vi "Test Case, Master Record.vi"() -> ()   [LabVIEW 2010]
panel:
  in  "Table Control":string[][](table)
  out "error out":errorcluster
  in  "error in":errorcluster
  in  "Initialize":bool=TRUE
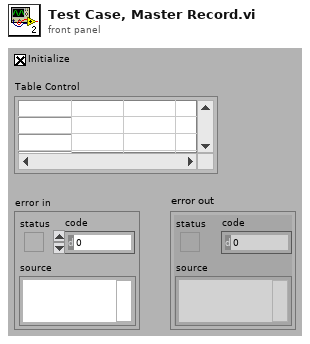
[diagram p1: front panel]
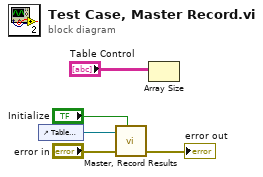
[diagram p0: block diagram]
diagram:
  n1 = control-ref of="Table Control"() -> (w1:refnum<vi>)
  n2 = call "Master, Record Results.vi"("Initialize (F)"="Initialize", "error in"="error in", "Tbl Refnum"=w1) -> ("error out"=→"error out":errorcluster)  [unwired: 7 in, 1 out]
  n3 = Array Size(array="Table Control") -> ()  [unwired: 1 out]
